vi "Init CAN TDMS Info.vi"(8 "error in (no error)":errorcluster, 9 "timestamp":timestamp, 10 "CAN frame":T1 {"type" items=["CAN Data", "CAN Remote"]; "identifier" format="%.0x"}, 11 "tdms file":refnum<k34>) -> (0 "error out":errorcluster, 3 "tdms file out":refnum<k34>)   [LabVIEW 2014]
uses:
  Global Data.vi
  <vilib>/Utility/tdmsutil.llb/TDMS Create Scaling Information (Linear).vi
  <vilib>/RioEmbeddedCAN/RioEmbeddedCAN.llb/CANFrameControl.ctl
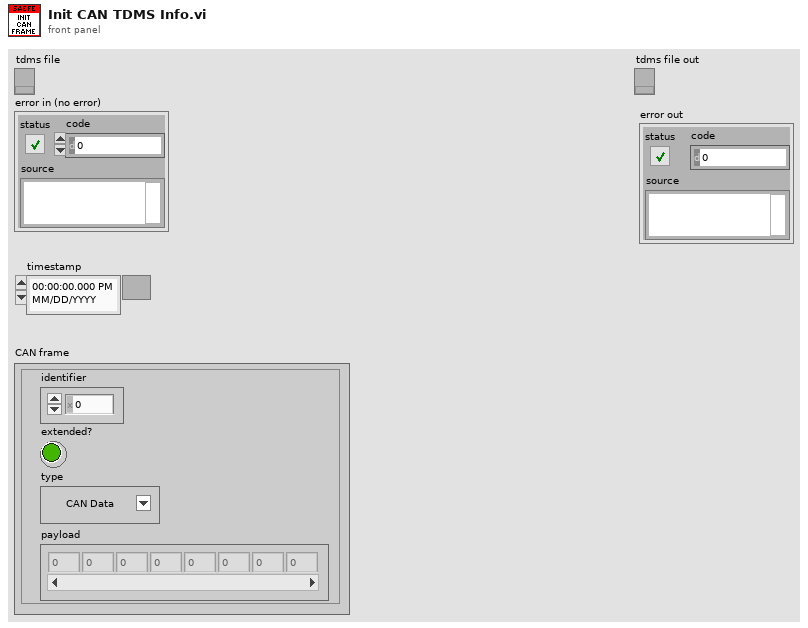
[diagram p1: front panel]
types:
  T1 = typedef "CANFrameControl.ctl" = cluster{"identifier":u32, "extended?":bool, "type":u8, "payload":u8[]}
  T2 = cluster{"slope":dbl, "y intercept":dbl, "input source":i32}
  T3 = cluster{"slope":dbl, "y intercept":dbl, "input source":i32}[]
  T4 = enum16{"Off", "On, Not Charging", "Charging", "Charging Finished", "Charging Error"}
  T5 = enum16{"Disconnected", "Pre-charging", "Main Charging", "Balancing", "Charging Finished OK", "Charging Error"}
  T6 = typedef "BMS Telemetry.ctl" = cluster{"Ignition":bool, "Charger Mains":bool, "Fast Charge":bool, "Simple Charger Enabled":bool, "Car State":enum16{"Off", "On, Not Charging", "Charging", "Charging Finished", "Charging Error"}, "Charging State":enum16{"Disconnected", "Pre-charging", "Main Charging", "Balancing", "Charging Finished OK", "Charging Error"}, "Charging Stage Duration":u16, "Last Charging Error":enum16{"No Error", "Cell Voltage Too Low", "No Comm from Cells so can't start", "Maximum charging stage duration expired", "No Comm from Cels so can't balande", "Cannot set balancing voltage", "Cell temps too high", "No Comms so can't determine temp", "# of Cells Mismatch", "Cells Overvoltage", "Cell Protection Event occured."}, "Number of Detected Cells":u8, "Under-Voltage":bool, "Over-Voltage":bool, "Overheat":bool, "Leakage":bool, "No Cell Comms":bool, "Low Voltage":bool, "High Temperature":bool, "Min Cell V":dbl, "Max Cell V":dbl, "Mean Cell V":dbl, "Total V":dbl, "Min Cell t":dbl, "Max Cell t":dbl, "Mean Cell t":dbl, "Cell Voltages":cluster{"[0]":dbl, "[1]":dbl, "[2]":dbl, "[3]":dbl, "[4]":dbl, "[5]":dbl, "[6]":dbl, "[7]":dbl, "[8]":dbl, "[9]":dbl, "[10]":dbl, "[11]":dbl, "[12]":dbl, "[13]":dbl, "[14]":dbl, "[15]":dbl, "[16]":dbl, "[17]":dbl, "[18]":dbl, "[19]":dbl, "[20]":dbl, "[21]":dbl, "[22]":dbl, "[23]":dbl, "[24]":dbl, "[25]":dbl, "[26]":dbl, "[27]":dbl, "[28]":dbl, "[29]":dbl, "[30]":dbl, "[31]":dbl, "[32]":dbl, "[33]":dbl, "[34]":dbl, "[35]":dbl, "[36]":dbl, "[37]":dbl, "[38]":dbl, "[39]":dbl, "[40]":dbl, "[41]":dbl, "[42]":dbl, "[43]":dbl, "[44]":dbl, "[45]":dbl, "[46]":dbl, "[47]":dbl, "[48]":dbl, "[49]":dbl, "[50]":dbl, "[51]":dbl, "[52]":dbl, "[53]":dbl, "[54]":dbl, "[55]":dbl, "[56]":dbl, "[57]":dbl, "[58]":dbl, "[59]":dbl, "[60]":dbl, "[61]":dbl, "[62]":dbl, "[63]":dbl, "[64]":dbl, "[65]":dbl, "[66]":dbl, "[67]":dbl, "[68]":dbl, "[69]":dbl, "[70]":dbl}, "Cell Temps":cluster{"[0]":dbl, "[1]":dbl, "[2]":dbl, "[3]":dbl, "[4]":dbl, "[5]":dbl, "[6]":dbl, "[7]":dbl, "[8]":dbl, "[9]":dbl, "[10]":dbl, "[11]":dbl, "[12]":dbl, "[13]":dbl, "[14]":dbl, "[15]":dbl, "[16]":dbl, "[17]":dbl, "[18]":dbl, "[19]":dbl, "[20]":dbl, "[21]":dbl, "[22]":dbl, "[23]":dbl, "[24]":dbl, "[25]":dbl, "[26]":dbl, "[27]":dbl, "[28]":dbl, "[29]":dbl, "[30]":dbl, "[31]":dbl, "[32]":dbl, "[33]":dbl, "[34]":dbl, "[35]":dbl, "[36]":dbl, "[37]":dbl, "[38]":dbl, "[39]":dbl, "[40]":dbl, "[41]":dbl, "[42]":dbl, "[43]":dbl, "[44]":dbl, "[45]":dbl, "[46]":dbl, "[47]":dbl, "[48]":dbl, "[49]":dbl, "[50]":dbl, "[51]":dbl, "[52]":dbl, "[53]":dbl, "[54]":dbl, "[55]":dbl, "[56]":dbl, "[57]":dbl, "[58]":dbl, "[59]":dbl, "[60]":dbl, "[61]":dbl, "[62]":dbl, "[63]":dbl, "[64]":dbl, "[65]":dbl, "[66]":dbl, "[67]":dbl, "[68]":dbl, "[69]":dbl, "[70]":dbl}}
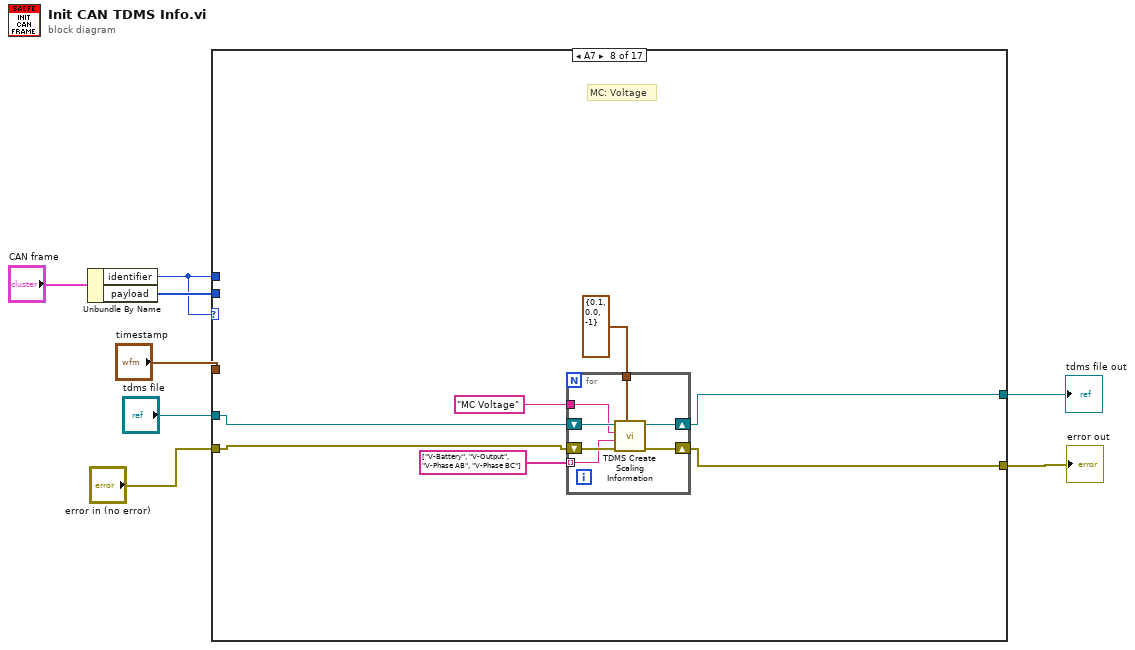
[diagram p0: block diagram]
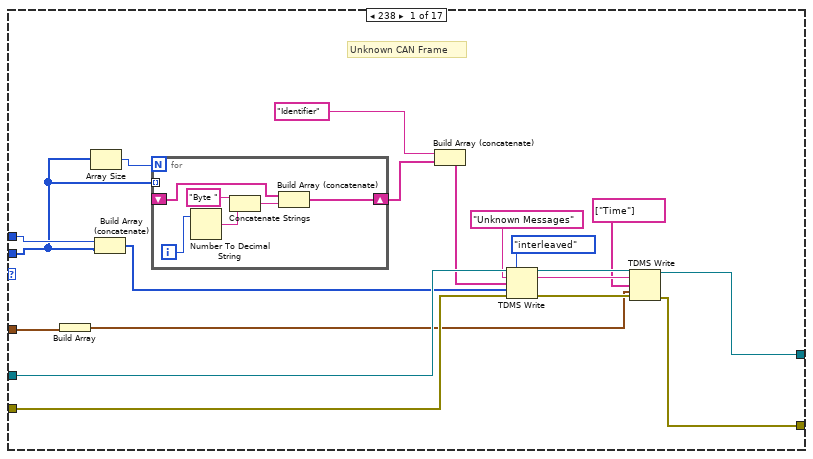
[diagram p2: hidden frame]
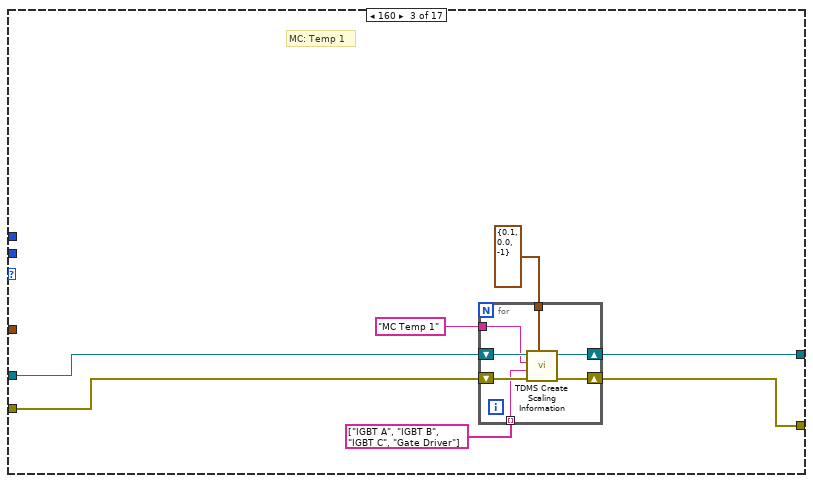
[diagram p4: hidden frame]
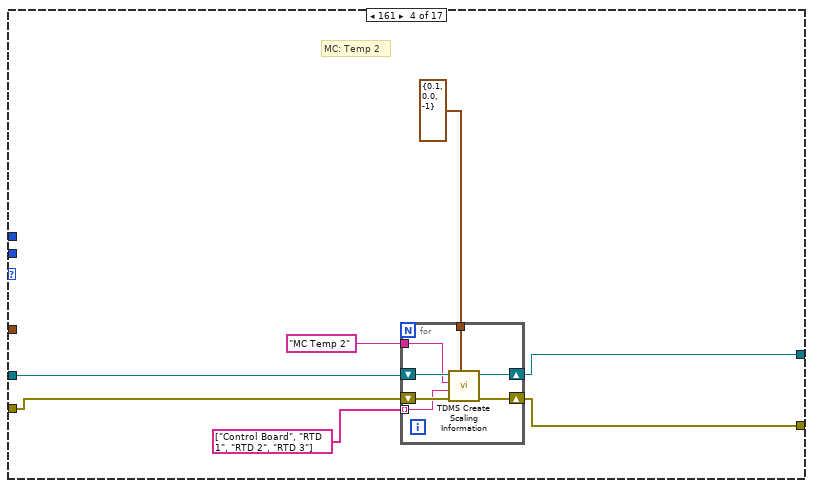
[diagram p5: hidden frame]
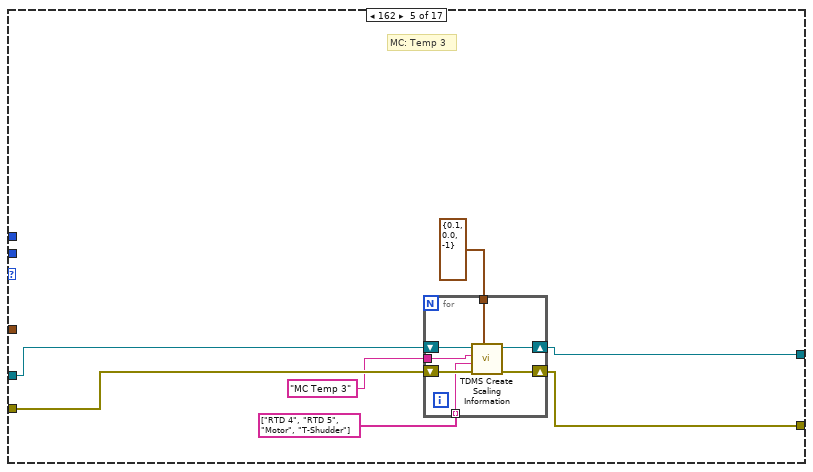
[diagram p6: hidden frame]
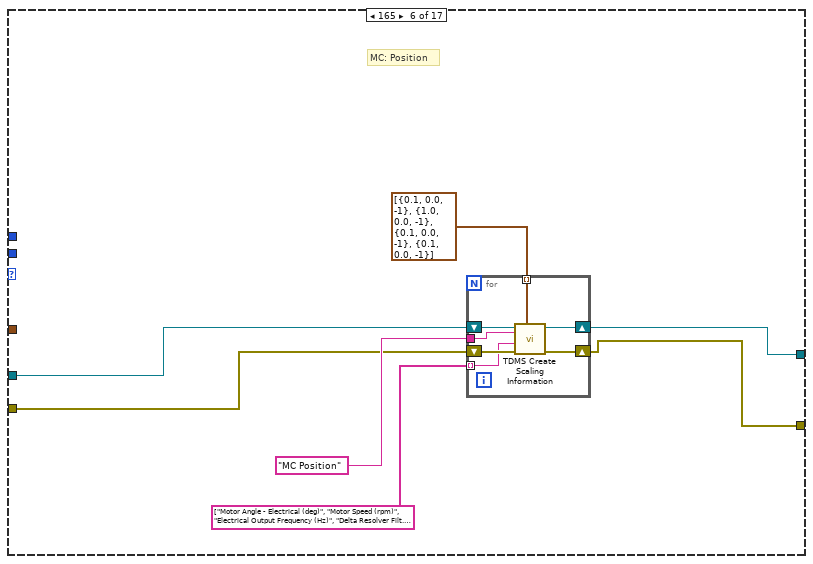
[diagram p7: hidden frame]
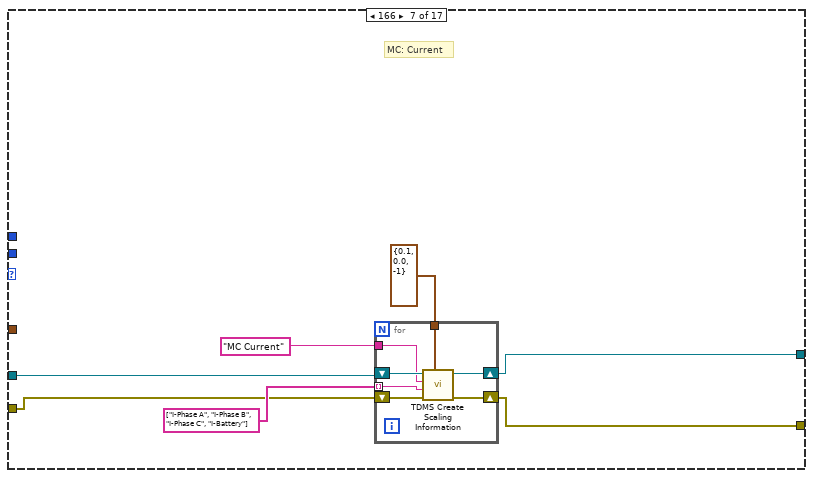
[diagram p8: hidden frame]
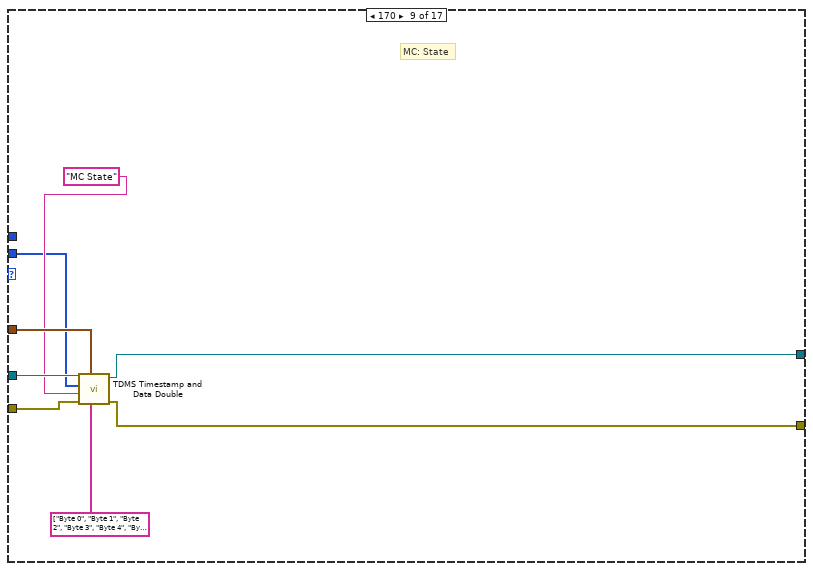
[diagram p9: hidden frame]
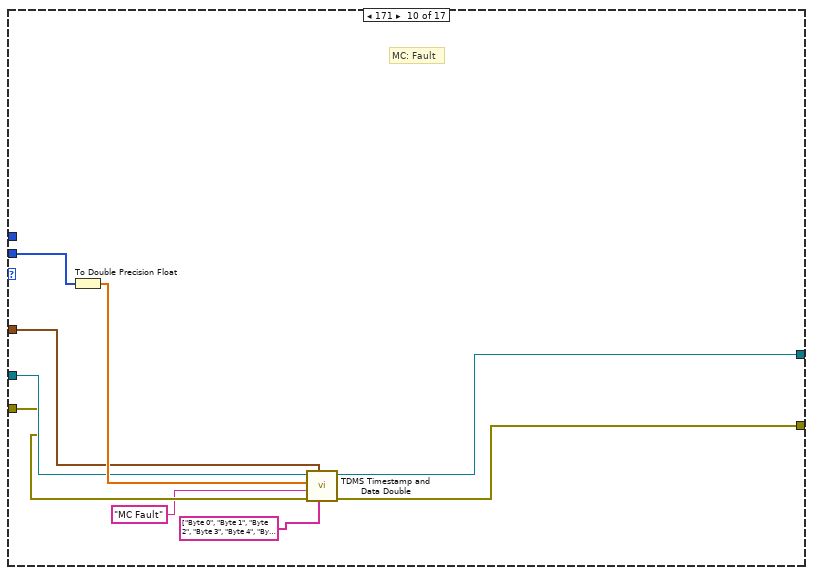
[diagram p10: hidden frame]
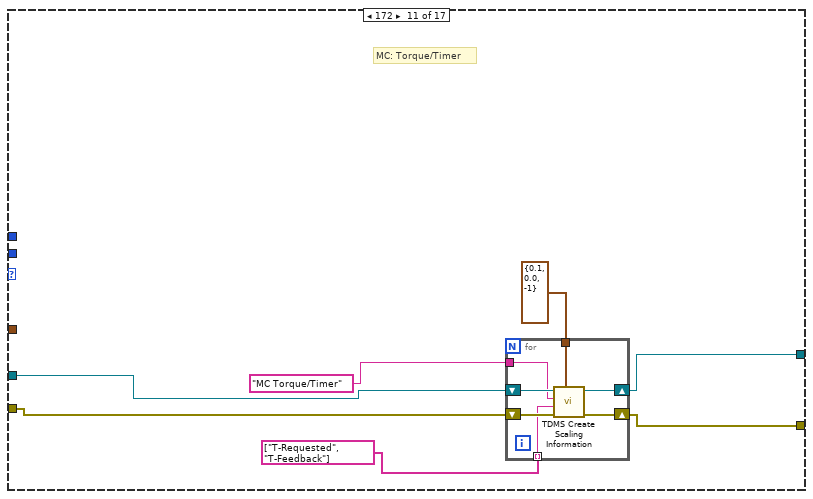
[diagram p11: hidden frame]
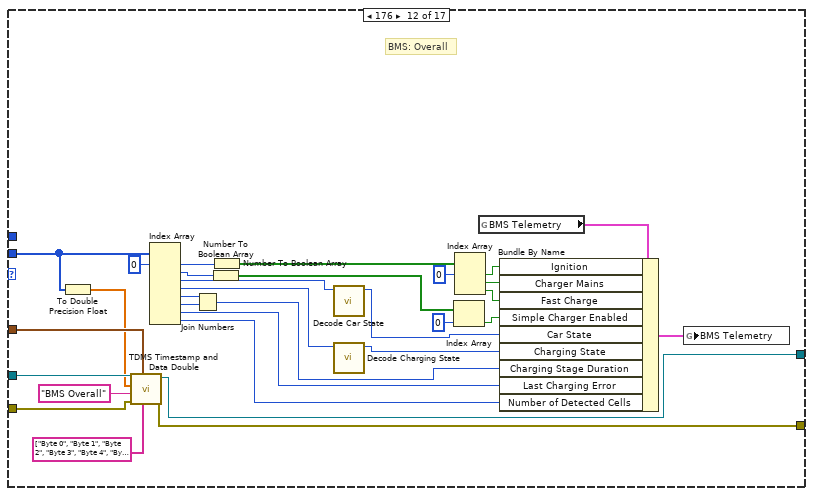
[diagram p12: hidden frame]
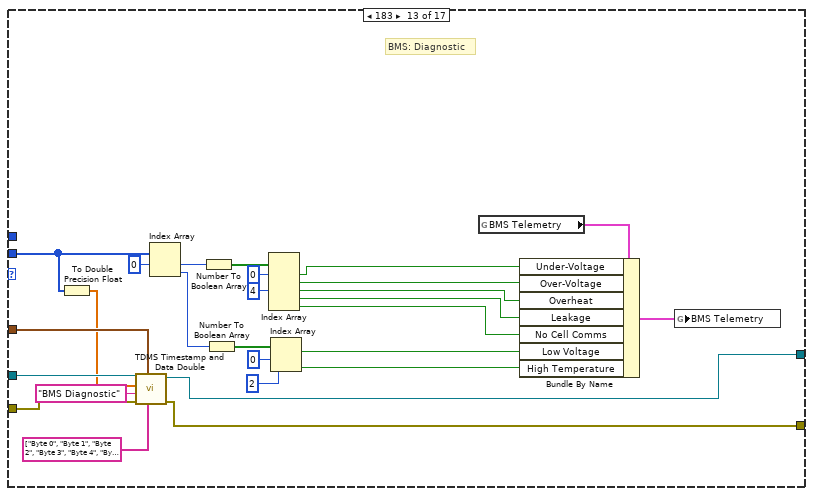
[diagram p13: hidden frame]
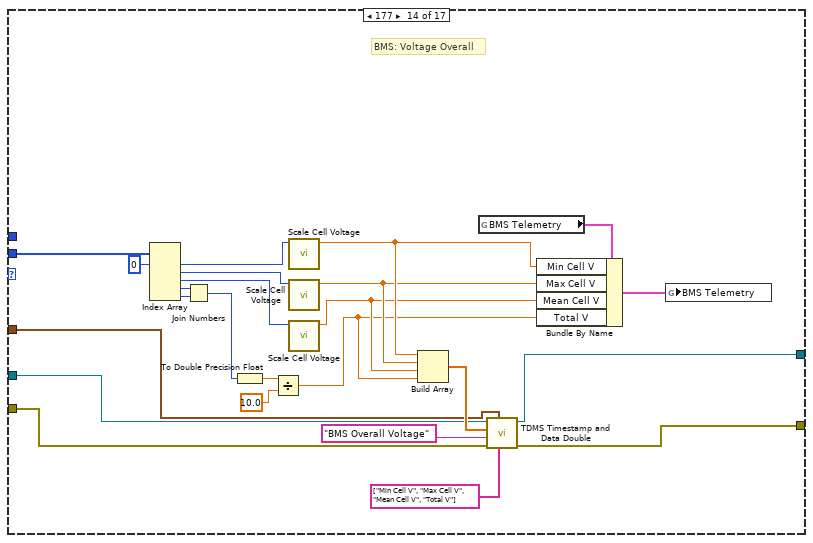
[diagram p14: hidden frame]
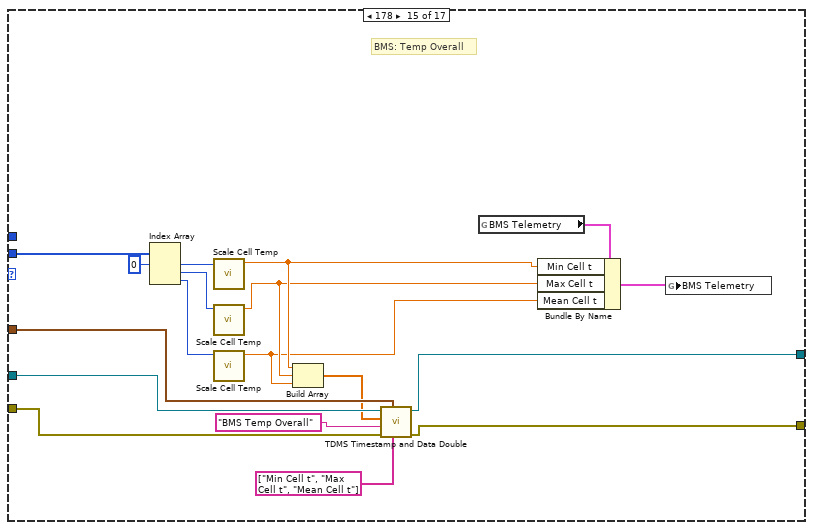
[diagram p15: hidden frame]
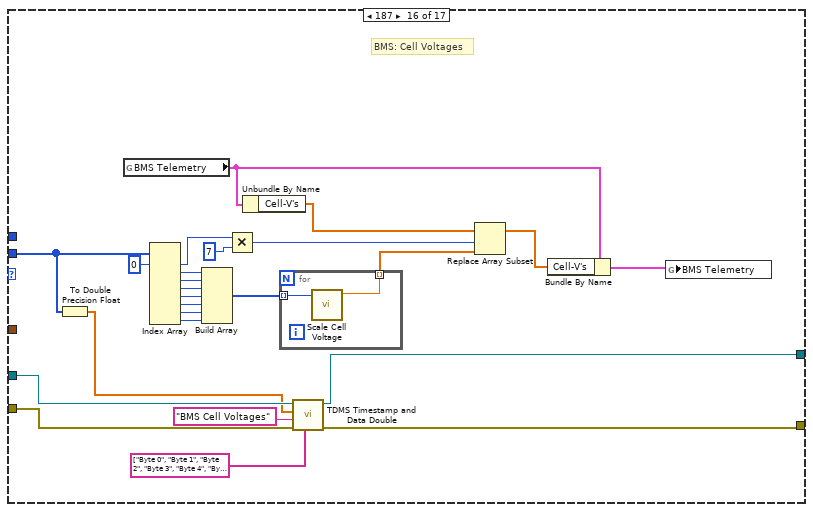
[diagram p16: hidden frame]
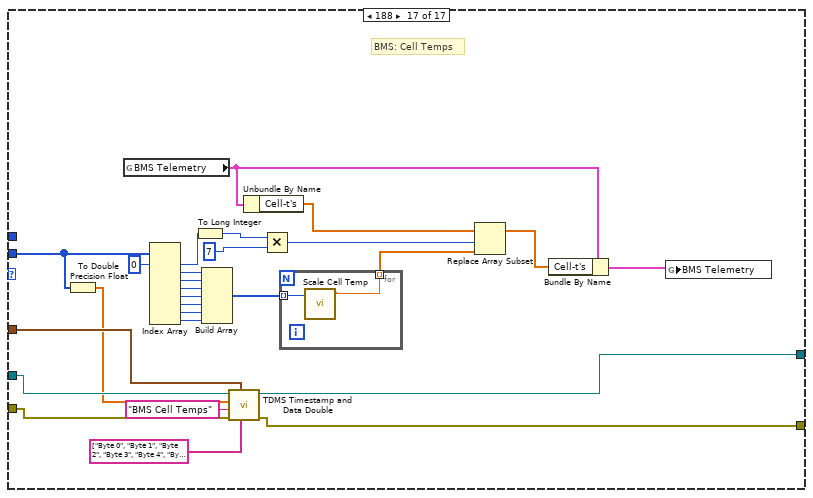
[diagram p17: hidden frame]
diagram:
  n1 = Unbundle By Name("CAN frame") -> ("identifier"=w5:u32, "payload"=w7:u8[])
  n2 = case shown="A7" w5 {
    tunnel: w5 -> [w27 _ _ _ _ _ _ _ _ _ _ _ _ _ _ _ _]
    tunnel: w7 -> [w9 _ _ _ _ _ _ _ w122 w136 _ w156 w187 w230 w248 w252 w283]
    tunnel: "timestamp" -> [w14 _ _ _ _ _ _ _ w127 w133 _ w157 w188 w213 w243 _ w288]
    tunnel: "tdms file" -> [w26 w35 w42 w55 w69 w81 w95 w109 w126 w134 w140 w159 w190 w215 w242 w258 w287]
    tunnel: [w11 w35 w41 w53 w65 w79 w93 w107 w121 w130 w138 w153 w184 w211 w234 w255 w284] -> w3
    tunnel: "error in (no error)" -> [w25 w34 w39 w54 w68 w80 w94 w108 w125 w132 w139 w158 w189 w214 w241 w257 w286]
    tunnel: [w12 w34 w40 w52 w64 w78 w92 w106 w120 w129 w137 w152 w183 w210 w233 w254 w285] -> w1
    frame 238 {
      # "Unknown CAN Frame"
      n3 = Build Array(w14) -> (w13:timestamp[])
      n4 = Array Size(array=w9) -> (size(s)=w10:i32)
      n5 = Build Array (concatenate)(w27, w9) -> (w24:u32[])
      n6 = for {
        N: w10 -> [_]
        tunnel: w9 -> [_] mode=indexing
        shift-right: [w32] -> w23
        shift-left: _ -> [w28]
        i -> [w31]
        n7 = Number To Decimal String(number=w31) -> (decimal integer string=w30:string)  [unwired: 1 in]
        n8 = Concatenate Strings("Byte " ("string"), w30) -> (w33:string)
        n9 = Build Array (concatenate)(w28, w33) -> (w32:string[])
      }
      n10 = Build Array (concatenate)("Identifier", w23) -> (w21:string[])
      n11 = TDMS Write(0:w26, 1:enum16{"decimated", "interleaved"}."interleaved" ("data layout (0:decimated)"), 5:"Unknown Messages" ("group name in (Untitled)"), 7:w21, 9:w24, 11:w25) -> (4:w18:refnum<k34>, 6:w16:string, 15:w17:errorcluster)  [unwired: 1 out]
      n12 = TDMS Write(0:w18, 5:w16, 7:string[] ["Time"] ("channel name(s) in (Untitled)"), 9:w13, 11:w17) -> (4:w11:refnum<k34>, 15:w12:errorcluster)  [unwired: 1 in, 2 out]
    }
    frame 0, Default {
      # "Do nothing for NULL frame"
    }
    frame 160 {
      # "MC: Temp 1"
      n13 = for {
        tunnel: "MC Temp 1" ("group name in (Untitled)") -> [w45]
        shift-right: [w48] -> w41
        shift-left: w42 -> [w49]
        shift-right: [w47] -> w40
        shift-left: w39 -> [w46]
        tunnel: string[] ["IGBT A", "IGBT B", "IGBT C", "Gate Driver"] ("channel name(s) in (Untitled)") -> [w44] mode=indexing
        tunnel: T2 {"slope"=0.1, "y intercept"=0.0, "input source"=-1} ("linear scale") -> [w43]
        n14 = call-poly <vilib>:"TDMS Create Scaling Information.vi"("linear scale"=w43, "error in (no error)"=w46, "channel name"=w44, "group name"=w45, "tdms file"=w49) -> ("error out"=w47:errorcluster, "tdms file out"=w48:refnum<k34>)  [unwired: 2 in, 3 out]
      }
    }
    frame 161 {
      # "MC: Temp 2"
      n15 = for {
        shift-right: [w62] -> w53
        shift-left: w55 -> [w63]
        shift-right: [w61] -> w52
        shift-left: w54 -> [w60]
        tunnel: T2 {"slope"=0.1, "y intercept"=0.0, "input source"=-1} ("linear scale") -> [w59]
        tunnel: string[] ["Control Board", "RTD 1", "RTD 2", "RTD 3"] ("channel name(s) in (Untitled)") -> [w58] mode=indexing
        tunnel: "MC Temp 2" ("group name in (Untitled)") -> [w57]
        n16 = call-poly <vilib>:"TDMS Create Scaling Information.vi"("linear scale"=w59, "error in (no error)"=w60, "channel name"=w58, "group name"=w57, "tdms file"=w63) -> ("error out"=w61:errorcluster, "tdms file out"=w62:refnum<k34>)  [unwired: 2 in, 3 out]
      }
    }
    frame 162 {
      # "MC: Temp 3"
      n17 = for {
        shift-right: [w76] -> w65
        shift-left: w69 -> [w77]
        shift-right: [w75] -> w64
        shift-left: w68 -> [w74]
        tunnel: T2 {"slope"=0.1, "y intercept"=0.0, "input source"=-1} ("linear scale") -> [w73]
        tunnel: "MC Temp 3" ("group name in (Untitled)") -> [w72]
        tunnel: string[] ["RTD 4", "RTD 5", "Motor", "T-Shudder"] ("channel name(s) in (Untitled)") -> [w71] mode=indexing
        n18 = call-poly <vilib>:"TDMS Create Scaling Information.vi"("linear scale"=w73, "error in (no error)"=w74, "channel name"=w71, "group name"=w72, "tdms file"=w77) -> ("error out"=w75:errorcluster, "tdms file out"=w76:refnum<k34>)  [unwired: 2 in, 3 out]
      }
    }
    frame 165 {
      # "MC: Position"
      n19 = for {
        shift-right: [w90] -> w79
        shift-left: w81 -> [w91]
        shift-right: [w89] -> w78
        shift-left: w80 -> [w88]
        tunnel: T3 [{"slope"=0.1, "y intercept"=0.0, "input source"=-1}, {"slope"=1.0, "y intercept"=0.0, "input source"=-1}, {"slope"=0.1, "y intercept"=0.0, "input source"=-1}, {"slope"=0.1, "y intercept"=0.0, "input source"=-1}] -> [w87] mode=indexing
        tunnel: "MC Position" ("group name in (Untitled)") -> [w86]
        tunnel: string[] ["Motor Angle - Electrical (deg)", "Motor Speed (rpm)", "Electrical Output Frequency (Hz)", "Delta Resolver Filt. (deg)"] ("channel name(s) in (Untitled)") -> [w85] mode=indexing
        n20 = call-poly <vilib>:"TDMS Create Scaling Information.vi"("linear scale"=w87, "error in (no error)"=w88, "channel name"=w85, "group name"=w86, "tdms file"=w91) -> ("error out"=w89:errorcluster, "tdms file out"=w90:refnum<k34>)  [unwired: 2 in, 3 out]
      }
    }
    frame 166 {
      # "MC: Current"
      n21 = for {
        tunnel: "MC Current" ("group name in (Untitled)") -> [w101]
        shift-right: [w104] -> w93
        shift-left: w95 -> [w105]
        shift-right: [w103] -> w92
        shift-left: w94 -> [w102]
        tunnel: T2 {"slope"=0.1, "y intercept"=0.0, "input source"=-1} ("linear scale") -> [w100]
        tunnel: string[] ["I-Phase A", "I-Phase B", "I-Phase C", "I-Battery"] ("channel name(s) in (Untitled)") -> [w99] mode=indexing
        n22 = call-poly <vilib>:"TDMS Create Scaling Information.vi"("linear scale"=w100, "error in (no error)"=w102, "channel name"=w99, "group name"=w101, "tdms file"=w105) -> ("error out"=w103:errorcluster, "tdms file out"=w104:refnum<k34>)  [unwired: 2 in, 3 out]
      }
    }
    frame 167 {
      # "MC: Voltage"
      n23 = for {
        shift-right: [w118] -> w107
        shift-left: w109 -> [w119]
        shift-right: [w117] -> w106
        shift-left: w108 -> [w116]
        tunnel: T2 {"slope"=0.1, "y intercept"=0.0, "input source"=-1} ("linear scale") -> [w115]
        tunnel: "MC Voltage" ("group name in (Untitled)") -> [w114]
        tunnel: string[] ["V-Battery", "V-Output", "V-Phase AB", "V-Phase BC"] ("channel name(s) in (Untitled)") -> [w113] mode=indexing
        n24 = call-poly <vilib>:"TDMS Create Scaling Information.vi"("linear scale"=w115, "error in (no error)"=w116, "channel name"=w113, "group name"=w114, "tdms file"=w119) -> ("error out"=w117:errorcluster, "tdms file out"=w118:refnum<k34>)  [unwired: 2 in, 3 out]
      }
    }
    frame 170 {
      # "MC: State"
      n25 = call "TDMS Timestamp and Data Double.vi"("channel name(s) in (Untitled)"=string[] ["Byte 0", "Byte 1", "Byte 2", "Byte 3", "Byte 4", "Byte 5", "Byte 6", "Byte 7"], "timestamp"=w127, "error in (no error)"=w125, "group name in (Untitled)"="MC State", "Array"=w122, "Refnum in"=w126) -> ("error out"=w120:errorcluster, "Refnum out"=w121:refnum<k34>)  [unwired: 4 in]
    }
    frame 171 {
      # "MC: Fault"
      n26 = To Double Precision Float(number=w136) -> (double precision float=w135:dbl[])
      n27 = call "TDMS Timestamp and Data Double.vi"("channel name(s) in (Untitled)"=string[] ["Byte 0", "Byte 1", "Byte 2", "Byte 3", "Byte 4", "Byte 5", "Byte 6", "Byte 7"], "timestamp"=w133, "error in (no error)"=w132, "group name in (Untitled)"="MC Fault", "Array"=w135, "Refnum in"=w134) -> ("error out"=w129:errorcluster, "Refnum out"=w130:refnum<k34>)  [unwired: 4 in]
    }
    frame 172 {
      # "MC: Torque/Timer"
      n28 = for {
        tunnel: "MC Torque/Timer" ("group name in (Untitled)") -> [w146]
        shift-right: [w149] -> w138
        shift-left: w140 -> [w150]
        shift-right: [w148] -> w137
        shift-left: w139 -> [w147]
        tunnel: string[] ["T-Requested", "T-Feedback"] ("channel name(s) in (Untitled)") -> [w145] mode=indexing
        tunnel: T2 {"slope"=0.1, "y intercept"=0.0, "input source"=-1} ("linear scale") -> [w144]
        n29 = call-poly <vilib>:"TDMS Create Scaling Information.vi"("linear scale"=w144, "error in (no error)"=w147, "channel name"=w145, "group name"=w146, "tdms file"=w150) -> ("error out"=w148:errorcluster, "tdms file out"=w149:refnum<k34>)  [unwired: 2 in, 3 out]
      }
    }
    frame 176 {
      # "BMS: Overall"
      n30 = To Double Precision Float(number=w156) -> (double precision float=w155:dbl[])
      n31 = call "TDMS Timestamp and Data Double.vi"("channel name(s) in (Untitled)"=string[] ["Byte 0", "Byte 1", "Byte 2", "Byte 3", "Byte 4", "Byte 5", "Byte 6", "Byte 7"], "timestamp"=w157, "error in (no error)"=w158, "group name in (Untitled)"="BMS Overall", "Array"=w155, "Refnum in"=w159) -> ("error out"=w152:errorcluster, "Refnum out"=w153:refnum<k34>)  [unwired: 4 in]
      n32 = Index Array(array=w156, index #1=0 ("index")) -> (element #1=w178:u8, element #2=w172:u8, element #3=w167:u8, element #4=w166:u8, element #5=w164:u8, element #6=w163:u8, element #7=w161:u8, element #8=w160:u8)  [unwired: 7 in]
      n33 = Join Numbers(hi=w164, lo=w163) -> ((hi.lo)=w162:u16)
      n34 = Number To Boolean Array(number=w172) -> (Boolean array=w170:bool[])
      n35 = Number To Boolean Array(number=w178) -> (Boolean array=w177:bool[])
      n36 = call "Decode Car State.vi"("Numeric"=w167) -> ("Car State"=w168:T4)  [unwired: 10 in]
      n37 = call "Decode Charging State.vi"("Numeric"=w166) -> ("Charging State"=w165:T5)  [unwired: 10 in]
      n38 = Index Array(array=w170, index=0) -> (element=w171:bool)
      n39 = Index Array(array=w177, index #1=0 ("index")) -> (element #1=w175:bool, element #2=w174:bool, element #3=w173:bool)  [unwired: 2 in]
      n40 = global read "Global Data.vi" "BMS Telemetry"() -> (w181:T6)
      n41 = Bundle By Name(cluster=w181, "Ignition"=w175, "Charger Mains"=w174, "Fast Charge"=w173, "Simple Charger Enabled"=w171, "Car State"=w168, "Charging State"=w165, "Charging Stage Duration"=w162, "Last Charging Error"=w161, "Number of Detected Cells"=w160) -> (w180:T6)
      n42 = global write "Global Data.vi" "BMS Telemetry"(w180) -> ()
    }
    frame 183 {
      # "BMS: Diagnostic"
      n43 = To Double Precision Float(number=w187) -> (double precision float=w186:dbl[])
      n44 = call "TDMS Timestamp and Data Double.vi"("channel name(s) in (Untitled)"=string[] ["Byte 0", "Byte 1", "Byte 2", "Byte 3", "Byte 4", "Byte 5", "Byte 6", "Byte 7"], "timestamp"=w188, "error in (no error)"=w189, "group name in (Untitled)"="BMS Diagnostic", "Array"=w186, "Refnum in"=w190) -> ("error out"=w183:errorcluster, "Refnum out"=w184:refnum<k34>)  [unwired: 4 in]
      n45 = Index Array(array=w187, index #1=0 ("index")) -> (element #1=w205:u8, element #2=w196:u8)  [unwired: 1 in]
      n46 = Number To Boolean Array(number=w205) -> (Boolean array=w204:bool[])
      n47 = Number To Boolean Array(number=w196) -> (Boolean array=w195:bool[])
      n48 = Index Array(array=w204, index #1=0 ("index"), index #3=4 ("index")) -> (element #1=w202:bool, element #2=w201:bool, element #3=w199:bool, element #4=w198:bool, element #5=w197:bool)  [unwired: 3 in]
      n49 = Index Array(array=w195, index #1=0 ("index"), index #2=2 ("index")) -> (element #1=w192:bool, element #2=w191:bool)
      n50 = global read "Global Data.vi" "BMS Telemetry"() -> (w208:T6)
      n51 = Bundle By Name(cluster=w208, "Under-Voltage"=w202, "Over-Voltage"=w201, "Overheat"=w199, "Leakage"=w198, "No Cell Comms"=w197, "Low Voltage"=w192, "High Temperature"=w191) -> (w207:T6)
      n52 = global write "Global Data.vi" "BMS Telemetry"(w207) -> ()
    }
    frame 177 {
      # "BMS: Voltage Overall"
      n53 = Index Array(array=w230, index #1=0 ("index")) -> (element #1=w228:u8, element #2=w227:u8, element #3=w226:u8, element #4=w225:u8, element #5=w224:u8)  [unwired: 4 in]
      n54 = Join Numbers(hi=w225, lo=w224) -> ((hi.lo)=w223:u16)
      n55 = To Double Precision Float(number=w223) -> (double precision float=w222:dbl)
      n56 = Divide(x=w222, y=10.0) -> (x/y=w217:dbl)
      n57 = call "Scale Cell Voltage.vi"("Numeric in"=w228) -> ("Numeric out"=w220:dbl)  [unwired: 10 in]
      n58 = call "Scale Cell Voltage.vi"("Numeric in"=w227) -> ("Numeric out"=w219:dbl)  [unwired: 10 in]
      n59 = call "Scale Cell Voltage.vi"("Numeric in"=w226) -> ("Numeric out"=w218:dbl)  [unwired: 10 in]
      n60 = Build Array(w220, w219, w218, w217) -> (w216:dbl[])
      n61 = global read "Global Data.vi" "BMS Telemetry"() -> (w232:T6)
      n62 = call "TDMS Timestamp and Data Double.vi"("channel name(s) in (Untitled)"=string[] ["Min Cell V", "Max Cell V", "Mean Cell V", "Total V"], "timestamp"=w213, "error in (no error)"=w214, "group name in (Untitled)"="BMS Overall Voltage", "Array"=w216, "Refnum in"=w215) -> ("error out"=w210:errorcluster, "Refnum out"=w211:refnum<k34>)  [unwired: 4 in]
      n63 = Bundle By Name(cluster=w232, "Min Cell V"=w220, "Max Cell V"=w219, "Mean Cell V"=w218, "Total V"=w217) -> (w231:T6)
      n64 = global write "Global Data.vi" "BMS Telemetry"(w231) -> ()
    }
    frame 178 {
      # "BMS: Temp Overall"
      n65 = Index Array(array=w248, index #1=0 ("index")) -> (element #1=w246:u8, element #2=w245:u8, element #3=w244:u8)  [unwired: 2 in]
      n66 = call "Scale Cell Temp.vi"("Numeric in"=w246) -> ("Numeric out"=w240:dbl)  [unwired: 10 in]
      n67 = call "Scale Cell Temp.vi"("Numeric in"=w245) -> ("Numeric out"=w239:dbl)  [unwired: 10 in]
      n68 = call "Scale Cell Temp.vi"("Numeric in"=w244) -> ("Numeric out"=w238:dbl)  [unwired: 10 in]
      n69 = Build Array(w240, w239, w238) -> (w237:dbl[])
      n70 = call "TDMS Timestamp and Data Double.vi"("channel name(s) in (Untitled)"=string[] ["Min Cell t", "Max Cell t", "Mean Cell t"], "timestamp"=w243, "error in (no error)"=w241, "group name in (Untitled)"="BMS Temp Overall", "Array"=w237, "Refnum in"=w242) -> ("error out"=w233:errorcluster, "Refnum out"=w234:refnum<k34>)  [unwired: 4 in]
      n71 = global read "Global Data.vi" "BMS Telemetry"() -> (w250:T6)
      n72 = Bundle By Name(cluster=w250, "Min Cell t"=w240, "Max Cell t"=w239, "Mean Cell t"=w238) -> (w249:T6)
      n73 = global write "Global Data.vi" "BMS Telemetry"(w249) -> ()
    }
    frame 187 {
      # "BMS: Cell Voltages"
      n74 = To Double Precision Float(number=w252) -> (double precision float=w251:dbl[])
      n75 = global read "Global Data.vi" "BMS Telemetry"() -> (w271:T6)
      n76 = Index Array(array=w252, index #1=0 ("index")) -> (element #1=w273:u8, element #2=w268:u8, element #3=w267:u8, element #4=w266:u8, element #5=w265:u8, element #6=w264:u8, element #7=w263:u8, element #8=w262:u8)  [unwired: 7 in]
      n77 = Build Array(w268, w267, w266, w265, w264, w263, w262) -> (w261:u8[])
      n78 = Multiply(x=w273, y=7) -> (x*y=w259:i32)
      n79 = Unbundle By Name(w271) -> ("Cell-V's"=w270:dbl[])
      n80 = for {
        tunnel: w261 -> [w277] mode=indexing
        tunnel: [w276] -> w260 mode=indexing
        n81 = call "Scale Cell Voltage.vi"("Numeric in"=w277) -> ("Numeric out"=w276:dbl)  [unwired: 10 in]
      }
      n82 = call "TDMS Timestamp and Data Double.vi"("channel name(s) in (Untitled)"=string[] ["Byte 0", "Byte 1", "Byte 2", "Byte 3", "Byte 4", "Byte 5", "Byte 6", "Byte 7"], "error in (no error)"=w257, "group name in (Untitled)"="BMS Cell Voltages", "Array"=w251, "Refnum in"=w258) -> ("error out"=w254:errorcluster, "Refnum out"=w255:refnum<k34>)  [unwired: 5 in]
      n83 = Replace Array Subset(array=w270, new element=w260, index=w259) -> (w269:dbl[])
      n84 = Bundle By Name(cluster=w271, "Cell-V's"=w269) -> (w275:T6)
      n85 = global write "Global Data.vi" "BMS Telemetry"(w275) -> ()
    }
    frame 188 {
      # "BMS: Cell Temps"
      n86 = To Double Precision Float(number=w283) -> (double precision float=w282:dbl[])
      n87 = global read "Global Data.vi" "BMS Telemetry"() -> (w301:T6)
      n88 = Index Array(array=w283, index #1=0 ("index")) -> (element #1=w278:u8, element #2=w298:u8, element #3=w297:u8, element #4=w296:u8, element #5=w295:u8, element #6=w294:u8, element #7=w293:u8, element #8=w292:u8)  [unwired: 7 in]
      n89 = To Long Integer(number=w278) -> (32bit integer=w279:i32)
      n90 = Build Array(w298, w297, w296, w295, w294, w293, w292) -> (w291:u8[])
      n91 = call "TDMS Timestamp and Data Double.vi"("channel name(s) in (Untitled)"=string[] ["Byte 0", "Byte 1", "Byte 2", "Byte 3", "Byte 4", "Byte 5", "Byte 6", "Byte 7"], "timestamp"=w288, "error in (no error)"=w286, "group name in (Untitled)"="BMS Cell Temps", "Array"=w282, "Refnum in"=w287) -> ("error out"=w285:errorcluster, "Refnum out"=w284:refnum<k34>)  [unwired: 4 in]
      n92 = Unbundle By Name(w301) -> ("Cell-t's"=w300:dbl[])
      n93 = Multiply(x=w279, y=7) -> (x*y=w289:i32)
      n94 = for {
        tunnel: w291 -> [w305] mode=indexing
        tunnel: [w306] -> w290 mode=indexing
        n95 = call "Scale Cell Temp.vi"("Numeric in"=w305) -> ("Numeric out"=w306:dbl)  [unwired: 10 in]
      }
      n96 = Replace Array Subset(array=w300, new element=w290, index=w289) -> (w299:dbl[])
      n97 = Bundle By Name(cluster=w301, "Cell-t's"=w299) -> (w304:T6)
      n98 = global write "Global Data.vi" "BMS Telemetry"(w304) -> ()
    }
  }
  "tdms file out" <- w3
  "error out" <- w1
